vi "Execute.vi"(8 "error in (no error)":errorcluster, 9 "System in":refnum<class "System.lvclass">, 10 "Command in":refnum<class "Command.lvclass">, 11 "GrabberArms-RetractingState in":refnum<class "GrabberArms-RetractingState.lvclass">) -> (0 "error out":errorcluster, 2 "Next State":refnum<class "State.lvclass">, 3 "GrabberArms-RetractingState out":refnum<class "GrabberArms-RetractingState.lvclass">)   [LabVIEW 2013, in "GrabberArms-RetractingState.lvclass"]
uses:
  GrabberArms-RetractingState.lvclass
  Commands/Command/Command.lvclass
  Systems/System/System.lvclass
  State/State.lvclass
  GA-Retracted-State/GrabberArms-RetractedState.lvclass
  Systems/GrabberArms/GrabberArms.lvclass
  Robot Global Data.vi
panel:
  in  "Wait time to retract":u32=3000
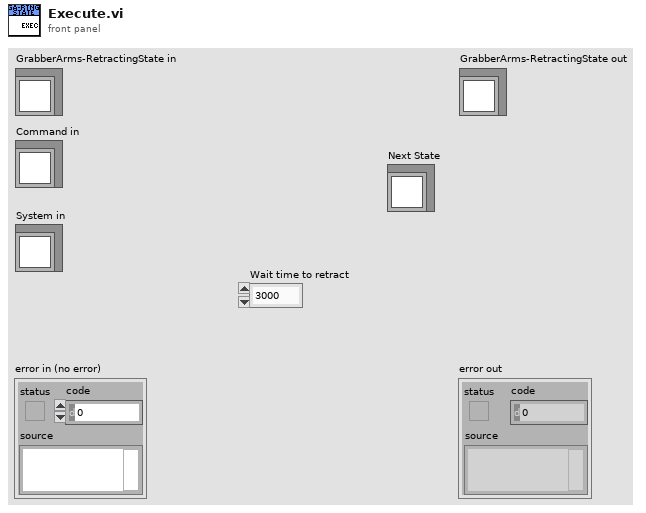
[diagram p1: front panel]
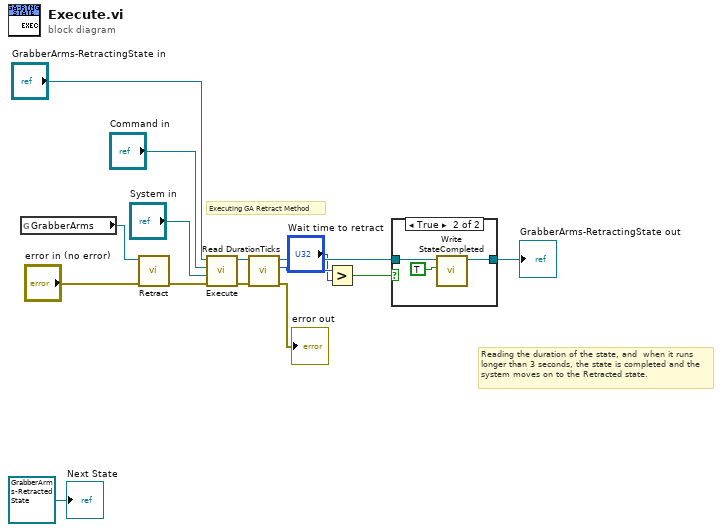
[diagram p0: block diagram]
diagram:
  # "Reading the duration of the state, and  when it runs longer than 3 seconds, the state is completed and the system moves on to the Retracted state."
  # "Executing GA Retract Method"
  n1 = global read "Robot Global Data.vi" "GrabberArms"() -> (w2:refnum<class "GrabberArms.lvclass">)
  n2 = call-dynamic "Retract.vi"("error in (no error)"="error in (no error)", "GrabberArms in"=w2) -> ("error out"=w13:errorcluster)  [unwired: 8 in, 1 out]
  n3 = call-parent "Execute.vi"("error in (no error)"=w13, "System in"="System in", "Command in"="Command in", "State in"="GrabberArms-RetractingState in") -> ("error out"=w7:errorcluster, "State out"=w12:refnum<class "GrabberArms-RetractingState.lvclass">)  [unwired: 5 in, 1 out]
  n4 = call "Read DurationTicks.vi"("error in (no error)"=w7, "State in"=w12) -> ("error out"=→"error out":errorcluster, "DurationTicks"=w10:u32, "State out"=w11:refnum<class "GrabberArms-RetractingState.lvclass">)  [unwired: 7 in]
  n5 = Greater?(x=w10, y="Wait time to retract") -> (0:w4:bool)
  n6 = case shown="True" w4 {
    tunnel: w11 -> [w16 w19]
    tunnel: [w16 w17] -> w8
    frame False {
    }
    frame True {
      n7 = call-dynamic "Write StateCompleted.vi"("StateCompleted"=TRUE, "State in"=w19) -> ("State out"=w17:refnum<class "GrabberArms-RetractingState.lvclass">)  [unwired: 8 in, 1 out]
    }
  }
  "GrabberArms-RetractingState out" <- w8
  "Next State" <- refnum<class "GrabberArms-RetractedState.lvclass"> refnum ("GrabberArms-RetractedState.lvclass")
